vi "Sensors Global Data.vi"() -> ()   [LabVIEW 2013]
panel:
  in  "Sensors Global Data":T1
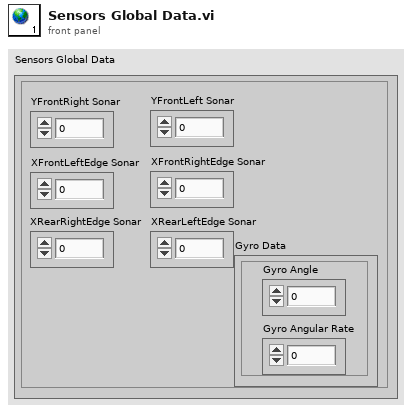
[diagram p1: front panel]
types:
  T1 = cluster{"YFrontRight Sonar":dbl, "YFrontLeft Sonar":dbl, "XFrontRightEdge Sonar":dbl, "XRearLeftEdge Sonar":dbl, "XFrontLeftEdge Sonar":dbl, "XRearRightEdge Sonar":dbl, "Gyro Data":cluster{"Gyro Angle":dbl, "Gyro Angular Rate":dbl}}
diagram:
